vi "Gen Ch List.vi"(11 "Prefix":string) -> (2 "Channel Names":string[](array[string])=["Telescope RA", "Telescope DEC", "Telescope Moving?", "Telescope Status"], 3 "Channel List":refnum<class "HK Item.lvclass">[](array[class]))   [LabVIEW 2022 SP3, in "Temp Control.lvclass"]
uses:
  Temp Control.lvclass
  hk-channel-class/hk-channel-class/HK Item/HK Item.lvclass
  hk-channel-class/hk-channel-class/HK Item/HK Channel Units and Setup.ctl
  hk-channel-class/hk-channel-class/HK Item/HK Channel enum Data Type.ctl
  Temp Control.lvclass/Temp Control.ctl
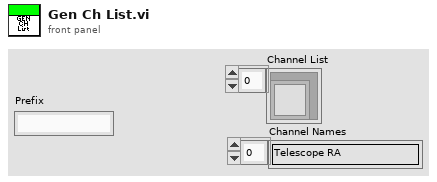
[diagram p1: front panel]
types:
  T1 = typedef "HK Item.lvclass/HK Channel Units and Setup.ctl" = cluster{"Unit Type":string, "Units":string, "Configuration":string, "Digits":i32, "Data Type":T2, "Exponential?":bool, "Source":string}
  T2 = typedef "HK Item.lvclass/HK Channel enum Data Type.ctl" = enum16{"Floating Point", "Integer", "Enum", "String", "Waveform", "File"}
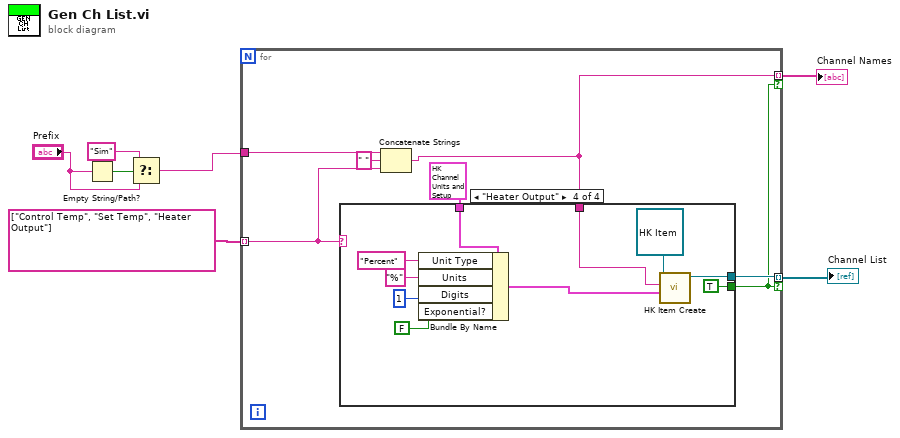
[diagram p0: block diagram]
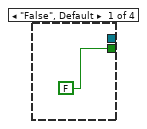
[diagram p2: hidden frame]
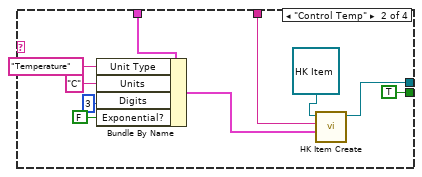
[diagram p3: hidden frame]
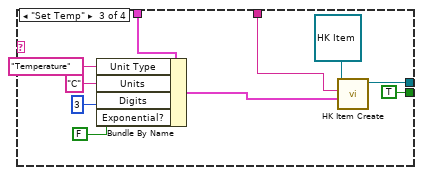
[diagram p4: hidden frame]
diagram:
  n1 = Empty String/Path?(string/path="Prefix") -> (empty?=w4:bool)
  n2 = Select(t="Sim", s=w4, f="Prefix") -> (s? t:f=w2:string)
  n3 = for {
    tunnel: string[] ["Control Temp", "Set Temp", "Heater Output"] -> [w12] mode=indexing
    tunnel: [w10] -> w5 mode=indexing if=w9
    tunnel: [w8] -> w6 mode=indexing if=w9
    tunnel: w2 -> [w13]
    n4 = Concatenate Strings(w13, " " ("string"), w12) -> (w8:string)
    n5 = case shown="\"Heater Output\"" w12 {
      tunnel: T1 {"Unit Type"="", "Units"="", "Configuration"="", "Digits"=3, "Data Type"=enum."Floating Point", "Exponential?"=FALSE, "Source"=""} ("Channel Setup") -> [_ w25 w35 w45]
      tunnel: w8 -> [_ w18 w29 w39]
      tunnel: [_ w17 w27 w37] -> w10
      tunnel: [FALSE TRUE TRUE TRUE] -> w9
      frame "False", Default {
      }
      frame "Control Temp" {
        n6 = Bundle By Name(cluster=w25, "Unit Type"="Temperature", "Units"="C", "Digits"=3, "Exponential?"=FALSE) -> (w19:T1)
        n7 = call-dynamic "HK Item Create.vi"("Channel Setup"=w19, "Name"=w18, "HK Item in"=refnum<class "HK Item.lvclass"> refnum) -> ("HK Item out"=w17:refnum<class "HK Item.lvclass">)  [unwired: 7 in, 1 out]
      }
      frame "Set Temp" {
        n8 = Bundle By Name(cluster=w35, "Unit Type"="Temperature", "Units"="C", "Digits"=3, "Exponential?"=FALSE) -> (w30:T1)
        n9 = call-dynamic "HK Item Create.vi"("Channel Setup"=w30, "Name"=w29, "HK Item in"=refnum<class "HK Item.lvclass"> refnum) -> ("HK Item out"=w27:refnum<class "HK Item.lvclass">)  [unwired: 7 in, 1 out]
      }
      frame "Heater Output" {
        n10 = Bundle By Name(cluster=w45, "Unit Type"="Percent", "Units"="%", "Digits"=1, "Exponential?"=FALSE) -> (w40:T1)
        n11 = call-dynamic "HK Item Create.vi"("Channel Setup"=w40, "Name"=w39, "HK Item in"=refnum<class "HK Item.lvclass"> refnum) -> ("HK Item out"=w37:refnum<class "HK Item.lvclass">)  [unwired: 7 in, 1 out]
      }
    }
  }
  "Channel List" <- w5
  "Channel Names" <- w6
